vi "Gamma_range.vi"(0 "Illuminant Table":string[][](array[string])) -> (1 "Interpolate":bool, 2 "In range?":bool, 3 "GammaInterval":dbl[](array[numeric]))   [LabVIEW 2013]
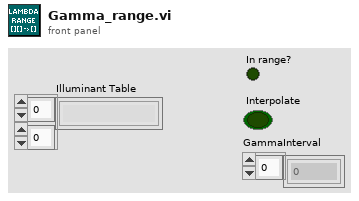
[diagram p1: front panel]
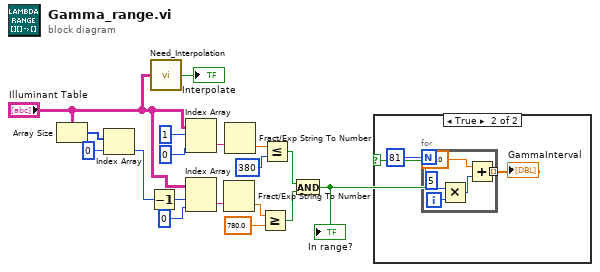
[diagram p0: block diagram]
diagram:
  n1 = Array Size(array="Illuminant Table") -> (size(s)=w5:i32[])
  n2 = Index Array(array=w5, index=0) -> (element=w3:i32)
  n3 = Decrement(x=w3) -> (x-1=w17:i32)
  n4 = call "Need_Interpolation.vi"("Illuminants"="Illuminant Table") -> ("Interpolate"=→"Interpolate":bool)
  n5 = Index Array(array="Illuminant Table", index (row)=1, index (col)=0) -> (element=w14:string)
  n6 = Index Array(array="Illuminant Table", index (row)=w17, index (col)=0 ("disabled index (col)")) -> (element=w13:string)
  n7 = Fract/Exp String To Number(string=w13) -> (number=w12:dbl)  [unwired: 3 in, 1 out]
  n8 = Fract/Exp String To Number(string=w14) -> (number=w9:dbl)  [unwired: 3 in, 1 out]
  n9 = Greater Or Equal?(x=w12, y=780.0) -> (x >= y?=w6:bool)
  n10 = Less Or Equal?(x=w9, y=380 ("x")) -> (x <= y?=w7:bool)
  n11 = And(x=w7, y=w6) -> (x .and. y?=w10:bool)
  "In range?" <- w10
  n12 = case shown="True" w10 {
    frame False {
    }
    frame True {
      n13 = for {
        N: 81 -> [_]
        tunnel: [w22] -> w20 mode=indexing
        i -> [w24]
        n14 = Multiply(x=5, y=w24) -> (x*y=w25:i32)
        n15 = Add(x=380.0, y=w25) -> (x+y=w22:dbl)
      }
      "GammaInterval" <- w20
    }
  }
